vi "统计字符串.vi"(1 "地图":i32[][](array[numeric])) -> (0 "字符串":string)   [LabVIEW 2017]
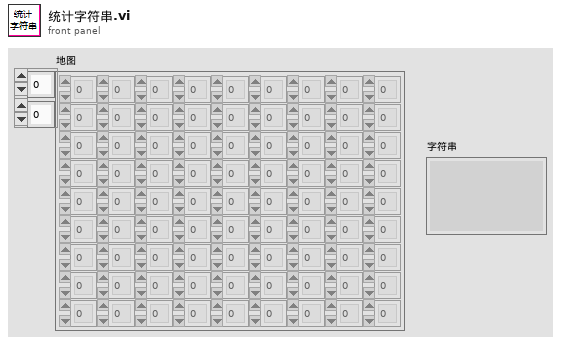
[diagram p1: front panel]
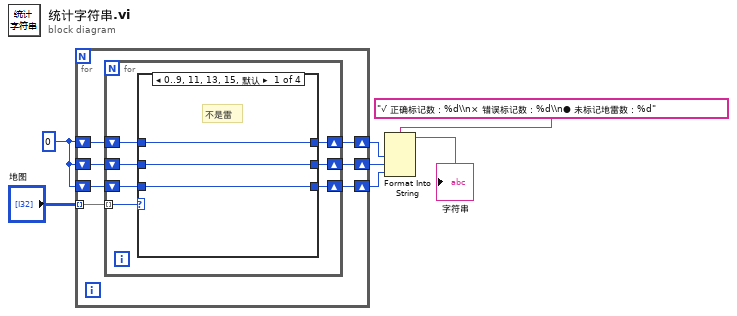
[diagram p0: block diagram]
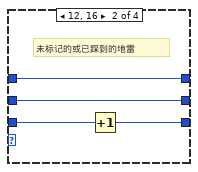
[diagram p2: hidden frame]
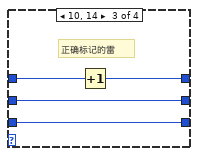
[diagram p3: hidden frame]
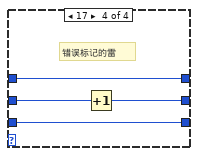
[diagram p4: hidden frame]
diagram:
  w6 = 0
  n1 = for {
    tunnel: "地图" -> [w14] mode=indexing
    shift-right: [w12] -> w2
    shift-left: w6 -> [w13]
    shift-right: [w8] -> w3
    shift-left: w6 -> [w11]
    shift-right: [w9] -> w1
    shift-left: w6 -> [w10]
    n2 = for {
      tunnel: w14 -> [w21] mode=indexing
      shift-right: [w19] -> w12
      shift-left: w13 -> [w20]
      shift-right: [w15] -> w8
      shift-left: w11 -> [w18]
      shift-right: [w16] -> w9
      shift-left: w10 -> [w17]
      n3 = case shown="0..9, 11, 13, 15, 默认" w21 {
        tunnel: w20 -> [w24 w28 w32 w33]
        tunnel: [w24 w28 w29 w33] -> w19
        tunnel: w18 -> [w23 w25 w31 w36]
        tunnel: w17 -> [w22 w27 w30 w34]
        tunnel: [w22 w26 w30 w34] -> w16
        tunnel: [w23 w25 w31 w35] -> w15
        frame 0..9, 11, 13, 15, Default {
          # "不是雷"
        }
        frame 12, 16 {
          # "未标记的或已踩到的地雷"
          n4 = Increment(x=w27) -> (x+1=w26:i32)
        }
        frame 10, 14 {
          # "正确标记的雷"
          n5 = Increment(x=w32) -> (x+1=w29:i32)
        }
        frame 17 {
          # "错误标记的雷"
          n6 = Increment(x=w36) -> (x+1=w35:i32)
        }
      }
    }
  }
  n7 = Format Into String(format string="√ 正确标记数：%d\\n× 错误标记数：%d\\n● 未标记地雷数：%d" ("格式字符串"), w2, w3, w1) -> (resulting string=→"字符串":string)  [unwired: 2 in, 1 out]
